vi "Examen.vi"() -> ()   [LabVIEW 2020]
uses:
  <vilib>/Instr/_visa.llb/VISA Configure Serial Port (Instr).vi
panel:
  out "Array":dbl[](array[numeric])
  out "Actual":dbl
  out "Mínimo":dbl
  out "Máximo":dbl
  out "Sensor & Filtro":i32(graph)
  out "Datos recibidos":string
  in  "stop":bool
  in  "Datos a enviar":string
  in  "Configuración UART":T1={"Puerto Arduino"="", "baud rate "=9600, "data bits"=8, "parity "=enum."None"} {"data bits" min=5 max=8 step=1}
  in  "Habilitar lectura":bool
  in  "Habilitar envío":bool
  # "Información lectura"
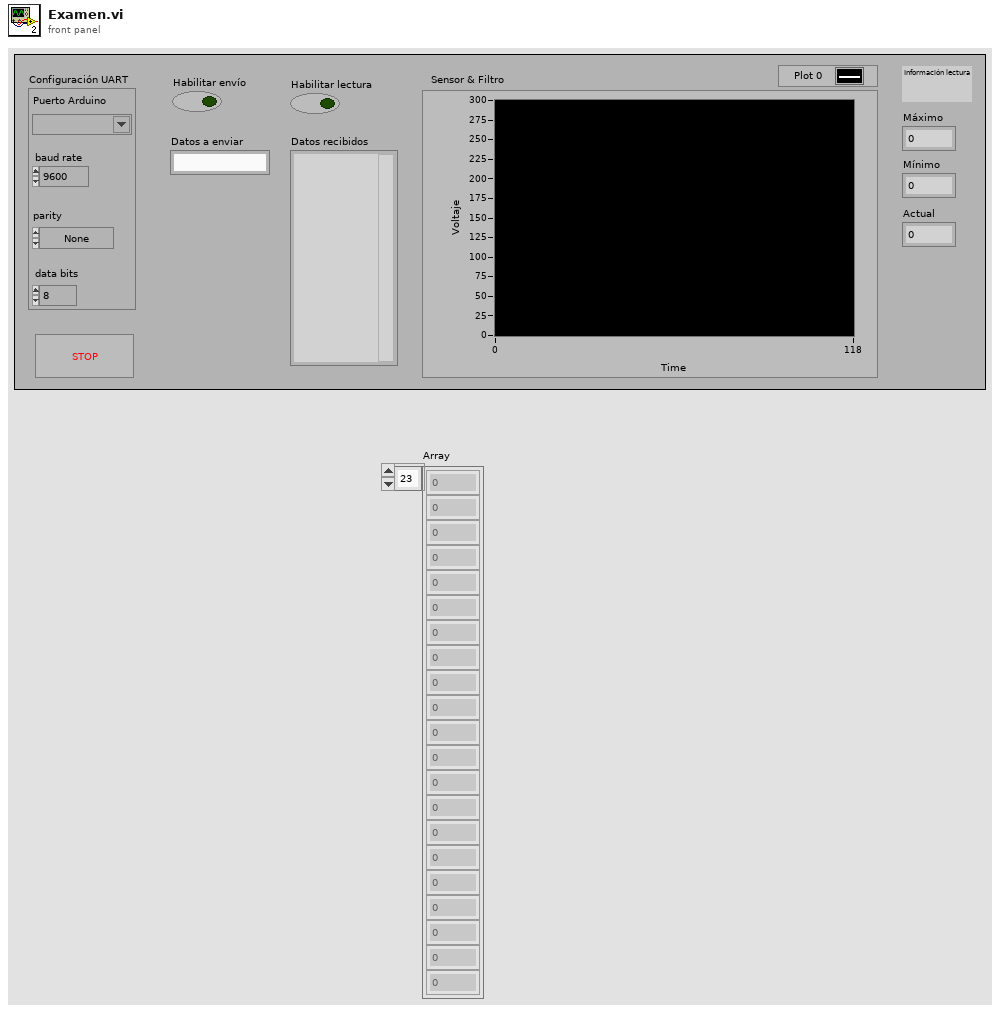
[diagram p1: front panel]
types:
  T1 = cluster{"Puerto Arduino":refnum<visa-resource-name>, "baud rate ":u32, "data bits":u16, "parity ":enum16{"None", "Odd", "Even", "Mark", "Space"}}
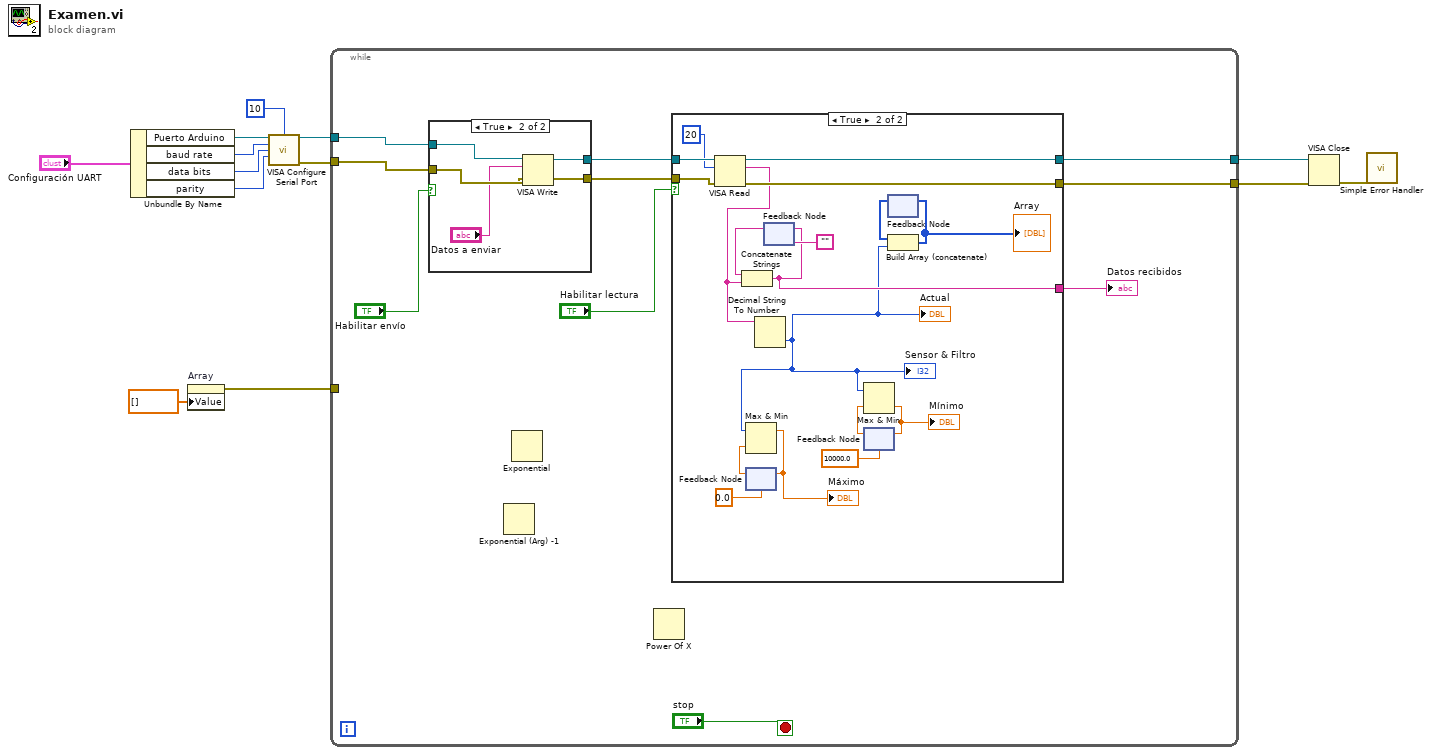
[diagram p0: block diagram]
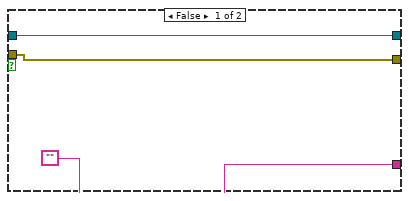
[diagram p2: hidden frame]
diagram:
  n1 = Unbundle By Name("Configuración UART") -> ("Puerto Arduino"=w7:refnum<visa-resource-name>, "baud rate"=w4:u32, "data bits"=w6:u16, "parity"=w5:enum16{"None", "Odd", "Even", "Mark", "Space"})
  n2 = property on="Array" class="Arr (strict)"("Value"=dbl[] [] ("Array")) -> (error out=w1:errorcluster)  [unwired: 2 in, 1 out]
  n3 = call-poly "VISA Configure Serial Port"("VISA resource name"=w7, "termination char\n(0xA = '\\n' = LF)"=u8 10 ("termination char\n(0xA = '\\n' = LF)"), "baud rate (9600)"=w4, "data bits (8)"=w6, "parity (0:none)"=w5) -> ("VISA resource name out"=w13:refnum<visa-resource-name>, "error out"=w12:errorcluster)  [unwired: 9 in]
  n4 = while {
    tunnel: w13 -> [w21]
    tunnel: w12 -> [w20]
    tunnel: [w17] -> w11
    tunnel: [w16] -> w10
    tunnel: w1 -> [_]
    stop <- "stop" stop-if-true
    n5 = case shown="True" "Habilitar envío" {
      tunnel: w21 -> [w46 w51]
      tunnel: w20 -> [w45 w50]
      tunnel: [w46 w49] -> w19
      tunnel: [w45 w48] -> w18
      frame False {
      }
      frame True {
        n6 = VISA Write(VISA resource name=w51, write buffer="Datos a enviar", error in (no error)=w50) -> (VISA resource name out=w49:refnum<visa-resource-name>, error out=w48:errorcluster)  [unwired: 1 out]
      }
    }
    n7 = Exponential (Arg) -1() -> ()  [unwired: 1 in, 1 out]
    n8 = Exponential() -> ()  [unwired: 1 in, 1 out]
    n9 = Power Of X() -> ()  [unwired: 2 in, 1 out]
    n10 = case shown="True" "Habilitar lectura" {
      tunnel: w19 -> [w26 w44]
      tunnel: w18 -> [w25 w43]
      tunnel: [w26 w42] -> w17
      tunnel: [w25 w41] -> w16
      tunnel: ["" w36] -> w14
      frame False {
      }
      frame True {
        n11 = VISA Read(VISA resource name=w44, byte count=u32 20, error in (no error)=w43) -> (VISA resource name out=w42:refnum<visa-resource-name>, read buffer=w37:string, error out=w41:errorcluster)  [unwired: 1 out]
        n12 = feedback #1(0.0) -> (w33:dbl)
        n13 = Decimal String To Number(string=w37) -> (number=w28:i32)  [unwired: 2 in, 1 out]
        "Sensor & Filtro" <- w28
        "Actual" <- w28
        n14 = Max & Min(x=w28, y=w33) -> (max(x,y)=w35:dbl)  [unwired: 1 out]
        "Máximo" <- w35
        n15 = feedback-in #1(w35) -> ()
        n16 = feedback #2("") -> (w39:string)
        n17 = Concatenate Strings "Concatenate Strings"(w39, w37) -> (w36:string)
        n18 = feedback-in #2(w36) -> ()
        n19 = feedback #3(10000.0) -> (w32:dbl)
        n20 = Max & Min(x=w28, y=w32) -> (min(x,y)=w34:dbl)  [unwired: 1 out]
        "Mínimo" <- w34
        n21 = feedback-in #3(w34) -> ()
        n22 = feedback #4() -> (w29:i32[])  [unwired: 1 in]
        n23 = Build Array (concatenate)(w29, w28) -> (w27:i32[])
        "Array" <- w27
        n24 = feedback-in #4(w27) -> ()
      }
    }
    "Datos recibidos" <- w14
  }
  n25 = VISA Close(VISA resource name=w11, error in (no error)=w10) -> (error out=w9:errorcluster)
  n26 = call <vilib>:"Simple Error Handler.vi"("error in (no error)"=w9) -> ()  [unwired: 4 in, 5 out]
